vi "API Tree.vi"   [LabVIEW 2019]
uses:
  src/Instrument.Lockin/Instrument.Lockin.lvclass
  e5681dd1-1a1a-4918-995b-862175d9f98f.vi
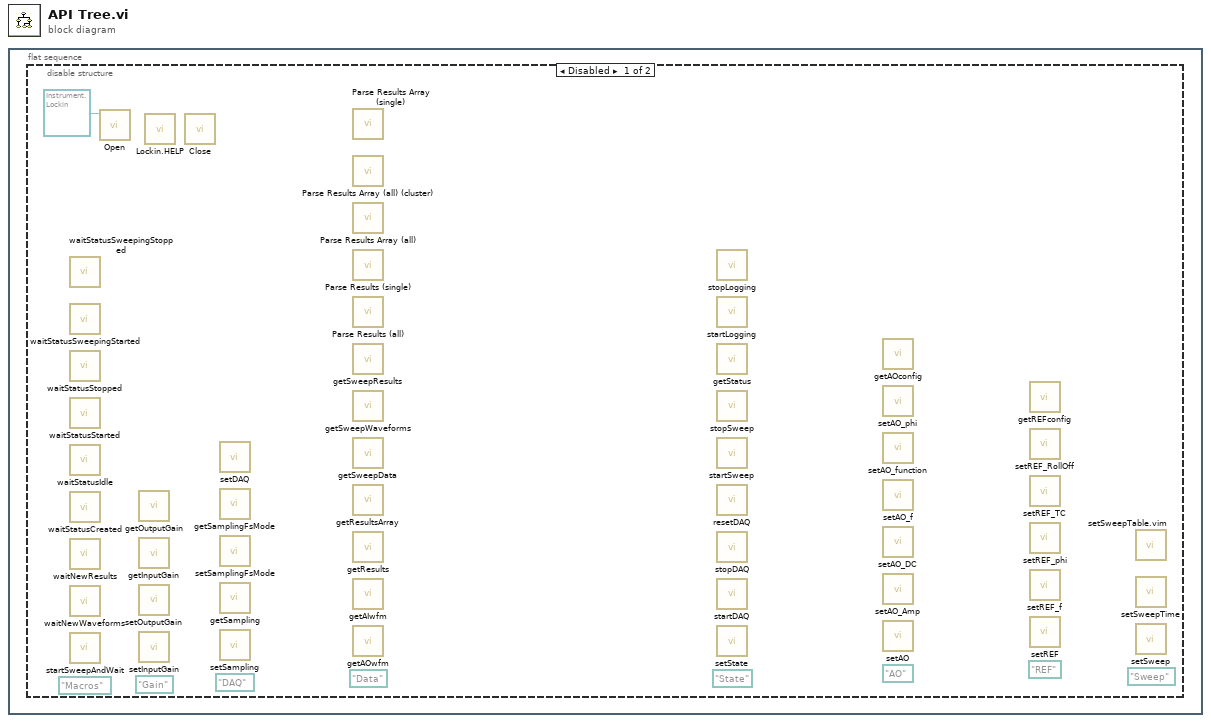
[diagram p0: block diagram]
diagram:
  n1 = flat-sequence {
    frame #0 {
      n2 = disable-structure shown="Disabled" {
        frame Disabled {
          (unwired) path "DAQ"
          (unwired) path "Gain"
          (unwired) path "Sweep"
          (unwired) path "REF"
          (unwired) path "AO"
          (unwired) path "State"
          (unwired) path "Data"
          (unwired) path "Macros"
          n3 = call-dynamic "waitStatusSweepingStopped.vi"() -> ()  [unwired: 10 in, 2 out]
          n4 = call-dynamic "waitStatusSweepingStarted.vi"() -> ()  [unwired: 10 in, 2 out]
          n5 = call-dynamic "waitStatusStopped.vi"() -> ()  [unwired: 10 in, 2 out]
          n6 = call-dynamic "waitStatusStarted.vi"() -> ()  [unwired: 10 in, 2 out]
          n7 = call-dynamic "waitStatusIdle.vi"() -> ()  [unwired: 10 in, 2 out]
          n8 = call-dynamic "waitStatusCreated.vi"() -> ()  [unwired: 10 in, 2 out]
          n9 = call-dynamic "waitNewResults.vi"() -> ()  [unwired: 9 in, 3 out]
          n10 = call-dynamic "waitNewWaveforms.vi"() -> ()  [unwired: 9 in, 3 out]
          n11 = call-dynamic "startSweepAndWait.vi"() -> ()  [unwired: 10 in, 2 out]
          n12 = call-dynamic "Open.vi"("Instrument.Lockin in"=refnum<class "Instrument.Lockin.lvclass"> refnum) -> ()  [unwired: 9 in, 2 out]
          n13 = call-dynamic "getOutputGain.vi"() -> ()  [unwired: 9 in, 3 out]
          n14 = call-dynamic "getInputGain.vi"() -> ()  [unwired: 9 in, 3 out]
          n15 = call-dynamic "setOutputGain.vi"() -> ()  [unwired: 10 in, 2 out]
          n16 = call-dynamic "setInputGain.vi"() -> ()  [unwired: 10 in, 2 out]
          n17 = call "Lockin.HELP.vi"() -> ()  [unwired: 9 in, 3 out]
          n18 = call-dynamic "Close.vi"() -> ()  [unwired: 10 in, 2 out]
          n19 = call-dynamic "setDAQ.vi"() -> ()  [unwired: 10 in, 2 out]
          n20 = call-dynamic "getSamplingFsMode.vi"() -> ()  [unwired: 9 in, 3 out]
          n21 = call-dynamic "setSamplingFsMode.vi"() -> ()  [unwired: 10 in, 2 out]
          n22 = call-dynamic "getSampling.vi"() -> ()  [unwired: 9 in, 3 out]
          n23 = call-dynamic "setSampling.vi"() -> ()  [unwired: 10 in, 2 out]
          n24 = call "Parse Results Array (single).vi"() -> ()  [unwired: 8 in, 4 out]
          n25 = call "Parse Results Array (all) (cluster).vi"() -> ()  [unwired: 8 in, 4 out]
          n26 = call "Parse Results Array (all).vi"() -> ()  [unwired: 8 in, 4 out]
          n27 = call "Parse Results (single).vi"() -> ()  [unwired: 8 in, 4 out]
          n28 = call "Parse Results (all).vi"() -> ()  [unwired: 8 in, 4 out]
          n29 = call-dynamic "getSweepResults.vi"() -> ()  [unwired: 8 in, 4 out]
          n30 = call-dynamic "getSweepWaveforms.vi"() -> ()  [unwired: 8 in, 4 out]
          n31 = call-dynamic "getSweepData.vi"() -> ()  [unwired: 9 in, 3 out]
          n32 = call-dynamic "getResultsArray.vi"() -> ()  [unwired: 8 in, 4 out]
          n33 = call-dynamic "getResults.vi"() -> ()  [unwired: 8 in, 4 out]
          n34 = call-dynamic "getAIwfm.vi"() -> ()  [unwired: 9 in, 3 out]
          n35 = call-dynamic "getAOwfm.vi"() -> ()  [unwired: 9 in, 3 out]
          n36 = call-dynamic "stopLogging.vi"() -> ()  [unwired: 10 in, 2 out]
          n37 = call-dynamic "startLogging.vi"() -> ()  [unwired: 10 in, 2 out]
          n38 = call-dynamic "getStatus.vi"() -> ()  [unwired: 9 in, 3 out]
          n39 = call-dynamic "stopSweep.vi"() -> ()  [unwired: 10 in, 2 out]
          n40 = call-dynamic "startSweep.vi"() -> ()  [unwired: 10 in, 2 out]
          n41 = call-dynamic "resetDAQ.vi"() -> ()  [unwired: 10 in, 2 out]
          n42 = call-dynamic "stopDAQ.vi"() -> ()  [unwired: 10 in, 2 out]
          n43 = call-dynamic "startDAQ.vi"() -> ()  [unwired: 10 in, 2 out]
          n44 = call-dynamic "setState.vi"() -> ()  [unwired: 10 in, 2 out]
          n45 = call-dynamic "getAOconfig.vi"() -> ()  [unwired: 9 in, 3 out]
          n46 = call-dynamic "setAO_phi.vi"() -> ()  [unwired: 10 in, 2 out]
          n47 = call-dynamic "setAO_function.vi"() -> ()  [unwired: 10 in, 2 out]
          n48 = call-dynamic "setAO_f.vi"() -> ()  [unwired: 10 in, 2 out]
          n49 = call-dynamic "setAO_DC.vi"() -> ()  [unwired: 10 in, 2 out]
          n50 = call-dynamic "setAO_Amp.vi"() -> ()  [unwired: 10 in, 2 out]
          n51 = call-dynamic "setAO.vi"() -> ()  [unwired: 10 in, 2 out]
          n52 = call-dynamic "getREFconfig.vi"() -> ()  [unwired: 9 in, 3 out]
          n53 = call-dynamic "setREF_RollOff.vi"() -> ()  [unwired: 10 in, 2 out]
          n54 = call-dynamic "setREF_TC.vi"() -> ()  [unwired: 10 in, 2 out]
          n55 = call-dynamic "setREF_phi.vi"() -> ()  [unwired: 10 in, 2 out]
          n56 = call-dynamic "setREF_f.vi"() -> ()  [unwired: 10 in, 2 out]
          n57 = call-dynamic "setREF.vi"() -> ()  [unwired: 10 in, 2 out]
          n58 = call "setSweepTable.vim"() -> ()  [unwired: 10 in, 2 out]
          n59 = call-dynamic "setSweepTime.vi"() -> ()  [unwired: 10 in, 2 out]
          n60 = call-dynamic "setSweep.vi"() -> ()  [unwired: 10 in, 2 out]
        }
        frame Enabled {
        }
      }
    }
  }
